vi "testReadNotifierServerStatus_tel.vi"(8 "error in (no error)":errorcluster) -> (0 "error out":errorcluster)   [LabVIEW 2018]
doc: "Test the readNotifierServerStatus.vi with tel selection."
uses:
  src/TcpServer/TcpServer.lvclass
  src/TcpServer/TcpServer.lvclass/TcpServer.ctl
  src/TcpServerBase/TcpServerBase.lvclass/TcpServerBase.ctl
  src/TcpServerTel/TcpServerTel.lvclass
  home/pcortes/Documents/github/ts_labview_tcp_json/src/TcpServerBase/TcpServerBase.lvclass
  <vilib>/addons/_JKI Toolkits/Caraya/classes/Assert/Assert Equal Type_Variant.vi
  <vilib>/addons/_JKI Toolkits/Caraya/classes/Test/Test.lvclass
  <vilib>/addons/_JKI Toolkits/Caraya/classes/Assert/Assert.lvclass
  src/TcpServerBase/TcpServerBase.lvclass
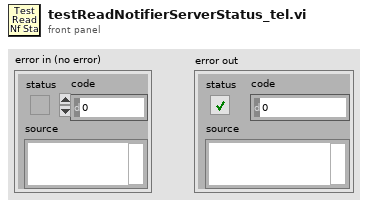
[diagram p1: front panel]
types:
  T1 = cluster{"connectionStatus":bool, "errorSource":string}
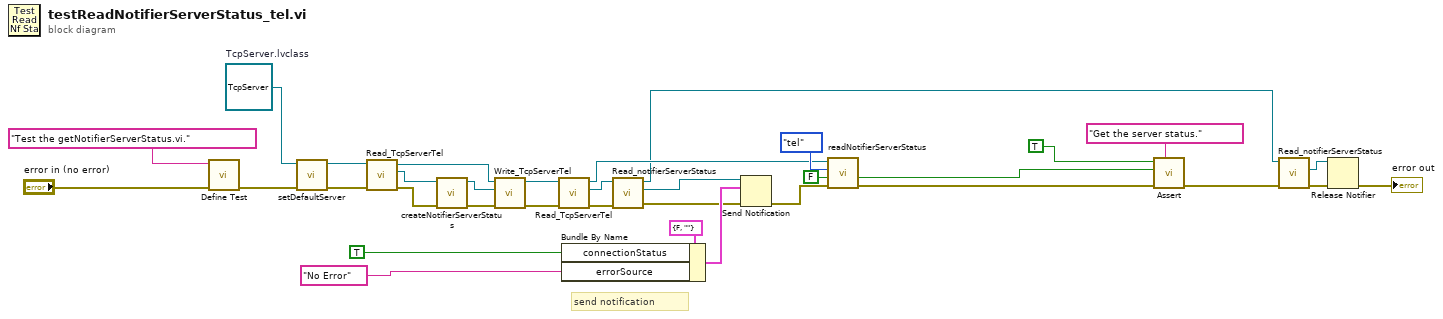
[diagram p0: block diagram]
diagram:
  w28 = refnum<class "TcpServer.lvclass"> refnum  # TcpServer.lvclass
  # "send notification"
  n1 = call <vilib>:"Define Test.vi"("error in (no error)"="error in (no error)", "Label (VI Title)"="Test the getNotifierServerStatus.vi.") -> ("error out"=w27:errorcluster)  [unwired: 9 in]
  n2 = call "setDefaultServer.vi"("error in (no error)"=w27, "TcpServer.lvclass"=w28) -> ("error out"=w26:errorcluster, "tcpServer out"=w25:refnum<class "TcpServer.lvclass">)  [unwired: 8 in]
  n3 = call "Read_TcpServerTel.vi"("error in (no error)"=w26, "TcpServer in"=w25) -> ("error out"=w24:errorcluster, "TcpServerTel.lvclass"=w12:refnum<class "TcpServerTel.lvclass">, "TcpServer out"=w10:refnum<class "TcpServer.lvclass">)  [unwired: 7 in]
  n4 = call "createNotifierServerStatus.vi"("error in (no error)"=w24, "tcpServerBase in"=w12) -> ("error out"=w13:errorcluster, "tcpServerBase out"=w9:refnum<class "TcpServerTel.lvclass">)  [unwired: 8 in]
  n5 = call "Write_TcpServerTel.vi"("error in (no error)"=w13, "TcpServerTel.lvclass"=w9, "TcpServer in"=w10) -> ("error out"=w11:errorcluster, "TcpServer out"=w7:refnum<class "TcpServer.lvclass">)  [unwired: 7 in]
  n6 = call "Read_TcpServerTel.vi"("error in (no error)"=w11, "TcpServer in"=w7) -> ("error out"=w8:errorcluster, "TcpServerTel.lvclass"=w5:refnum<class "TcpServerTel.lvclass">, "TcpServer out"=w6:refnum<class "TcpServer.lvclass">)  [unwired: 7 in]
  n7 = Bundle By Name(cluster=T1 {"connectionStatus"=FALSE, "errorSource"=""} ("notification"), "connectionStatus"=TRUE, "errorSource"="No Error" ("source")) -> (w19:T1)
  n8 = call "Read_notifierServerStatus.vi"("error in (no error)"=w8, "TcpServerBase in"=w5) -> ("error out"=w18:errorcluster, "notifierServerStatus"=w23:refnum<notifier>, "TcpServerBase out"=w4:refnum<class "TcpServerTel.lvclass">)  [unwired: 7 in]
  n9 = Send Notification(notification=w19, notifier=w23, error in (no error)=w18) -> (error out=w17:errorcluster)  [unwired: 1 out]
  n10 = call "readNotifierServerStatus.vi"("error in (no error)"=w17, "notifierStatusOld"=FALSE ("notification in"), "serverSelection"=enum16{"cmd", "tel"}."tel", "TcpServer in"=w6) -> ("error out (no error)"=w29:errorcluster, "notifierStatusNew"=w30:bool)  [unwired: 5 in, 1 out]
  n11 = call-poly <vilib>:"Assert.vi"("Label"="Get the server status.", "error in (no error)"=w29, "Y"=w30, "X"=TRUE) -> ("error out"=w31:errorcluster)  [unwired: 7 in]
  n12 = call "Read_notifierServerStatus.vi"("error in (no error)"=w31, "TcpServerBase in"=w4) -> ("error out"=w2:errorcluster, "notifierServerStatus"=w3:refnum<notifier>)  [unwired: 7 in, 1 out]
  n13 = Release Notifier(notifier=w3, error in (no error)=w2) -> (error out=→"error out":errorcluster)  [unwired: 1 in, 2 out]
